vi "BangBang_New.vi"(11 "Tolerance":dbl) -> (3 "BANG_BANG":T1 {"Measurment" format="%13.5p"; "Setpoint" format="%13.5p"; "Tolerance" format="%13.5p"})   [LabVIEW 2019, in "Trajectory_Library.lvlib"]
doc: "Implements a bang-bang controller, which outputs either 0 or 1 depending on whether the measurement is less than the setpoint. This maximally-aggressive control approach works very well for velocity control of high-inertia mechanisms, and poorly on most other things. \n \nNote that this is an *asymmetric* bang-bang controller - it will not exert any control effort in the reverse direction (e.g. it won't try to slow down an over-speeding shooter wheel). This asymmetry is *extremely important.* Bang-bang control is extremely simple, but also potentially hazardous. Always ensure that your motor controllers are set to \"coast\" before attempting to\ncontrol them with a bang-bang controller.\n\nCreates a new bang-bang controller.\n \nAlways ensure that your motor controllers are set to \"coast\" before attempting to control\nthem with a bang-bang controller.\n\nInputs:\n - Tolerance -- Tolerance for \"at setpoint\"\n\nOutputs:\n - BangBang -- Data cluster"
uses:
  Trajectory_Library.lvlib
  BANG_BANG.ctl
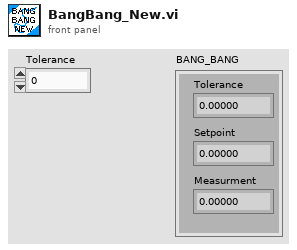
[diagram p1: front panel]
types:
  T1 = typedef "Trajectory_Library.lvlib/BANG_BANG.ctl" = cluster{"Tolerance":dbl, "Setpoint":dbl, "Measurment":dbl}
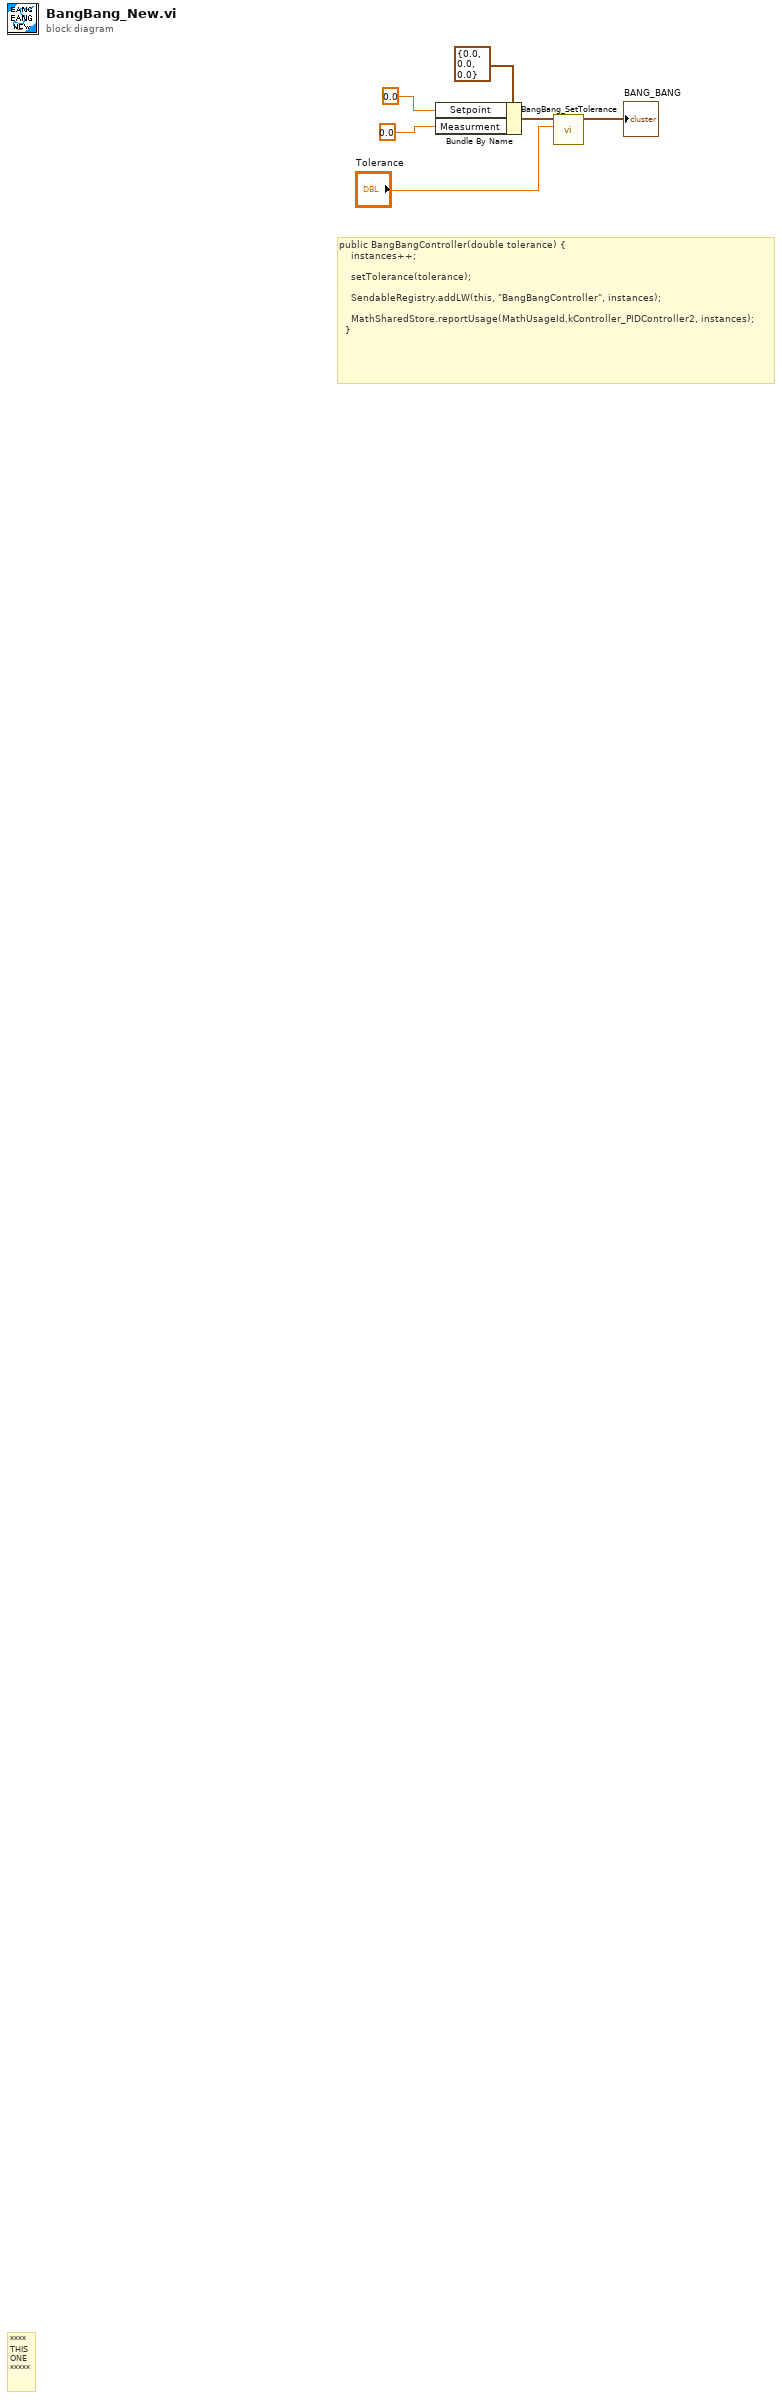
[diagram p0: block diagram]
diagram:
  # "public BangBangController(double tolerance) {\n    instances++;\n\n    setTolerance(tolerance);\n\n    SendableRegistry.addLW(this, \"BangBangController\", instances);\n\n    MathSharedStore.reportUsage(MathUsageId.kController_PIDController2, instances);\n  }"
  # "****\nTHIS\nONE\n*****"
  n1 = Bundle By Name(cluster=T1 {"Tolerance"=0.0, "Setpoint"=0.0, "Measurment"=0.0} ("BANG_BANG"), "Setpoint"=0.0, "Measurment"=0.0 ("Setpoint")) -> (w6:T1)
  n2 = call "BangBang_SetTolerance.vi"("Tolerance"="Tolerance", "BANG_BANG"=w6) -> ("out BANG_BANG"=→"BANG_BANG":T1)  [unwired: 9 in]
